vi "Format Text Style.vi"(4 "Text Color (Unchanged)":u32(colorbox), 6 "BG Color (Unchanged)":u32(colorbox), 7 "Table Cell? (F)":bool, 8 "Error in":errorcluster caption="Error in (no error)", 10 "Text Alignment (Left)":T1="left", 11 "String":string) -> (0 "Error out":errorcluster, 3 "Formatted Text":string)   [LabVIEW 2023, in "Confluence Formatting.lvlib"]
uses:
  Confluence Formatting.lvlib
  Types/Text Alignment Combo Box.ctl
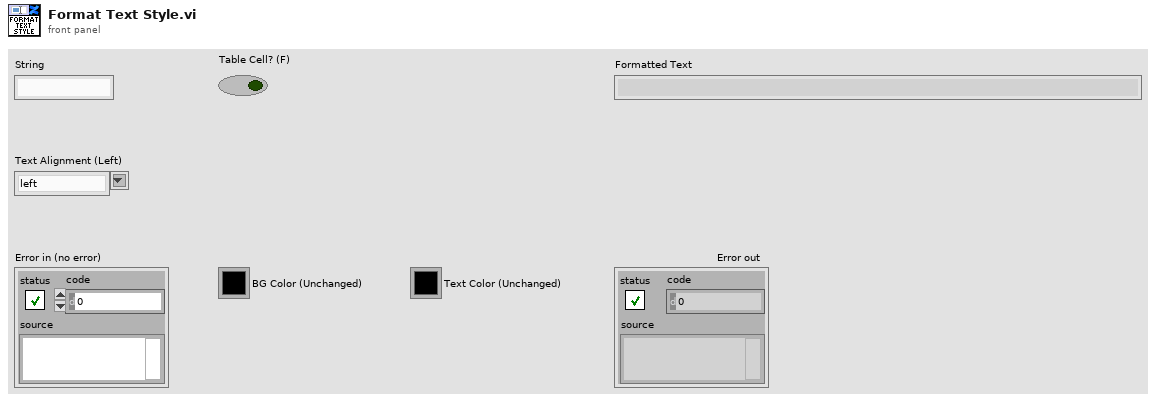
[diagram p1: front panel]
types:
  T1 = typedef "Confluence Formatting.lvlib/Text Alignment Combo Box.ctl" = string
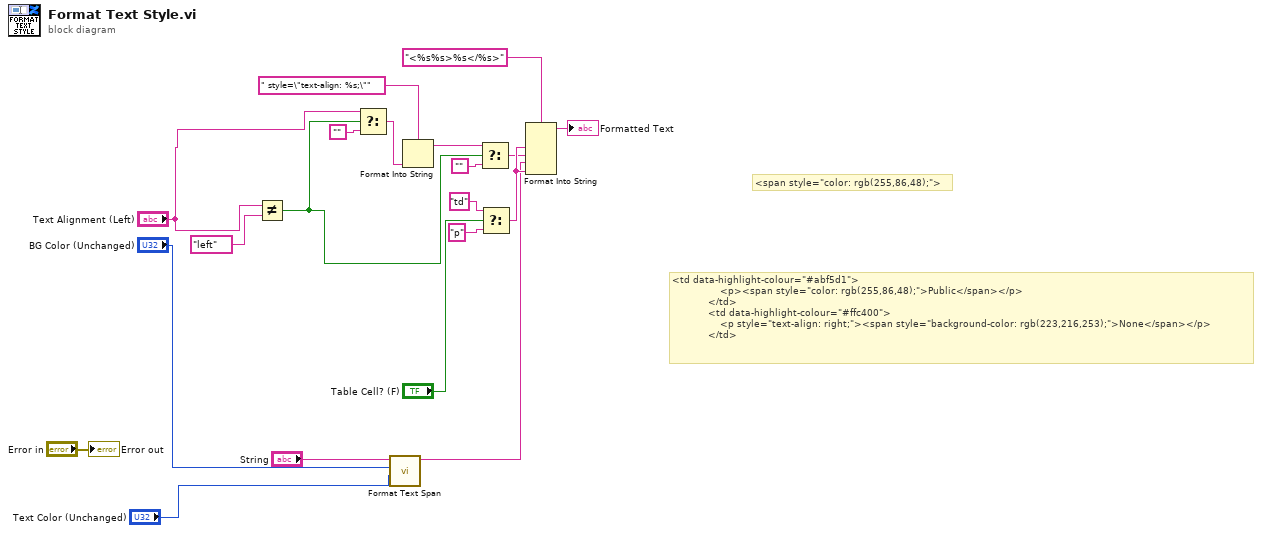
[diagram p0: block diagram]
diagram:
  # "<span style=\"color: rgb(255,86,48);\">"
  # "<td data-highlight-colour=\"#abf5d1\">\n                <p><span style=\"color: rgb(255,86,48);\">Public</span></p>\n            </td>\n            <td data-highlight-colour=\"#ffc400\">\n                <p style=\"text-align: right;\"><span style=\"background-color: rgb(223,216,253);\">None</span></p>\n            </td>"
  n1 = Not Equal?(x="Text Alignment (Left)", y=T1 "left") -> (x != y?=w2:bool)
  n2 = Select(t="Text Alignment (Left)", s=w2, f="") -> (s? t:f=w13:T1)
  n3 = call "Format Text Span.vi"("Text Color (Unchanged)"="Text Color (Unchanged)", "BG Color (Unchanged)"="BG Color (Unchanged)", "Text"="String") -> ("Formatted Span"=w5:string)  [unwired: 7 in, 1 out]
  n4 = Format Into String(format string=" style=\"text-align: %s;\"", w13) -> (resulting string=w12:string)  [unwired: 2 in, 1 out]
  n5 = Select(t=w12, s=w2, f="") -> (s? t:f=w9:string)
  n6 = Select(t="td", s="Table Cell? (F)", f="p") -> (s? t:f=w10:string)
  n7 = Format Into String(format string="<%s%s>%s</%s>", w10, w9, w5, w10) -> (resulting string=→"Formatted Text":string)  [unwired: 2 in, 1 out]
  "Error out" <- "Error in"
